vi "libssh2_knownhost_checkp - empty key - returns failure.vi"() -> ()   [LabVIEW 2013, in "libssh2_tests.lvlib"]
uses:
  libssh2_tests.lvlib
  libssh2/Knownhost Check Result.ctl
  libssh2/libssh2_init_default.vi
  <vilib>/addons/_JKI Toolkits/Caraya/classes/Assert/Assert Equal Value_Variant.vi
  <vilib>/addons/_JKI Toolkits/Caraya/classes/Test/Test.lvclass
  libssh2/libssh2.lvlib
  <vilib>/addons/_JKI Toolkits/Caraya/classes/Assert/Assert.lvclass
panel:
  out "error out":errorcluster
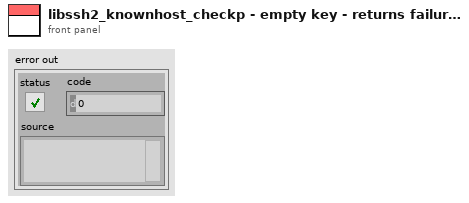
[diagram p1: front panel]
types:
  T1 = typedef "libssh2.lvlib/Knownhost Check Result.ctl" = enum16{"Match", "Mismatch", "Not Found", "Failure"}
  T2 = typedef "libssh2.lvlib/Session Refnum.ctl" = refnum<k1>
  T3 = typedef "libssh2.lvlib/Known Hosts Collection Refnum.ctl" = refnum<k1>
  T4 = typedef "libssh2.lvlib/Known Host Refnum.ctl" = refnum<k1>
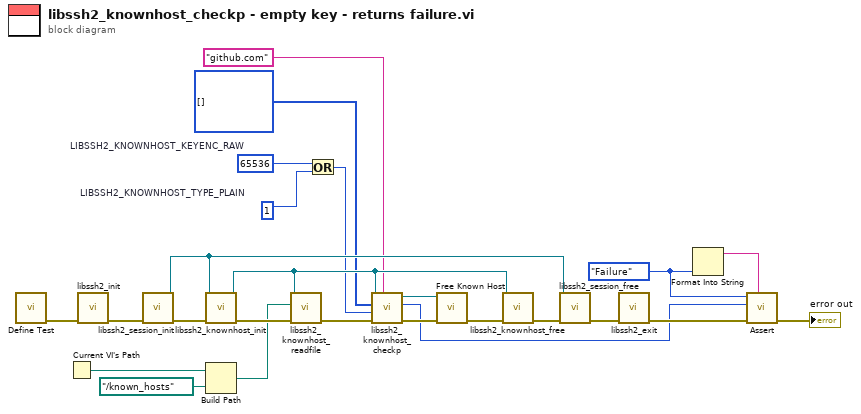
[diagram p0: block diagram]
diagram:
  w4 = Knownhost_Check_Result."Failure" ("result")
  w9 = 1  # LIBSSH2_KNOWNHOST_TYPE_PLAIN
  w10 = 65536  # LIBSSH2_KNOWNHOST_KEYENC_RAW
  n1 = call <vilib>:"Define Test.vi"() -> ("error out"=w24:errorcluster)  [unwired: 10 in, 1 out]
  n2 = Current VI's Path() -> (path=w15:path)
  n3 = call-poly "libssh2_init.vi"("error in (no error)"=w24) -> ("error out"=w23:errorcluster)  [unwired: 10 in]
  n4 = call "libssh2_session_init.vi"("error in (no error)"=w23) -> ("error out"=w22:errorcluster, "session"=w19:T2)  [unwired: 9 in]
  n5 = call "libssh2_knownhost_init.vi"("error in (no error)"=w22, "session"=w19) -> ("error out"=w17:errorcluster, "known hosts collection"=w11:T3)  [unwired: 8 in]
  n6 = Build Path(base path=w15, name or relative path=path "../known_hosts" ("filename")) -> (appended path=w13:path)
  n7 = call "libssh2_knownhost_readfile.vi"("error in (no error)"=w17, "filename"=w13, "known hosts collection"=w11) -> ("error out"=w16:errorcluster)  [unwired: 7 in, 1 out]
  n8 = Or(x=w10, y=w9) -> (x .or. y?=w8:i32)
  n9 = call "libssh2_knownhost_checkp.vi"("host"="github.com", "error in (no error)"=w16, "typemask"=w8, "key"=u8[] [] ("unsigned byte array"), "known hosts collection"=w11) -> ("error out"=w12:errorcluster, "result"=w5:T1, "known host"=w6:T4)  [unwired: 4 in]
  n10 = call "Free Known Host.vi"("error in (no error)"=w12, "known host"=w6) -> ("error out"=w7:errorcluster)  [unwired: 9 in]
  n11 = call "libssh2_knownhost_free.vi"("error in (no error)"=w7, "known hosts collection"=w11) -> ("error out"=w18:errorcluster)  [unwired: 9 in]
  n12 = call "libssh2_session_free.vi"("error in (no error)"=w18, "session"=w19) -> ("error out"=w21:errorcluster)  [unwired: 9 in]
  n13 = call "libssh2_exit.vi"("error in (no error)"=w21) -> ("error out"=w20:errorcluster)  [unwired: 10 in]
  n14 = Format Into String(w4) -> (resulting string=w3:string)  [unwired: 3 in, 1 out]
  n15 = call-poly <vilib>:"Assert.vi"("Label"=w3, "error in (no error)"=w20, "Y"=w5, "X"=w4) -> ("error out"=→"error out":errorcluster)  [unwired: 6 in, 1 out]
